vi "G# - CreatingAndDestroyingNamedObjects.vi"() -> ()   [LabVIEW 2020]
doc: "This example demonstrates how named objects work and also how objects behave if user counter is enabled.\n\nNaming Mode:\n1. Two objects with no names\n\nIf the object name is empty, a new object will always be created. User counter has no effect.\n\n2. Two objects with different names\n\nTwo objects are created with different name. There will be one user of each.\n\n3. Create and lookup object with equal names\n\nFirst a named object is created, then a new object with same name is attempted to be created, but since it already exists, the existing object with that name will be returned. If user counter is not enabled, create function will return error 400042. If user counter is enabled, the counter will be checked when trying to destroy the object and the object will not be destroyed until the last user of the object runs the destroy method."
uses:
  MyG#SubClass_class/MyG#SubClass.lvclass
  vi.lib/addons/_AddQ/G#Object/G#Object.lvclass
panel:
  out "# of objects killed":i32
  out "OK":bool
  in  "error in":errorcluster
  out "nr of users of the object":i32[](array[numeric])
  out "nr of objects of the class":i32[](array[numeric])
  in  "user counter":bool=TRUE
  in  "Naming mode":T1(ring)
  out "objects names":string[](array[string])
  out "error out":errorcluster
  # "This example demonstrates how named objects work and also how objects behave if user counter is enabled.\n\nNaming Mode:\n1. Two objects with no names\n\nIf the object name is empty, a new object will always be created. User counter has no effect.\n\n2. Two objects with different names\n\nTwo objects are created with different name. There will be one user of each.\n\n3. Create and lookup object with equal names\n\nFirst a named object is created, then a new object with same name is attempted to be created, but since it already exists, the existing object with that name will be returned. If user counter is not enabled, create function will return error 400042. If user counter is enabled, the counter will be checked when trying to destroy the object and the object will not be destroyed until the last user of the object runs the destroy method."
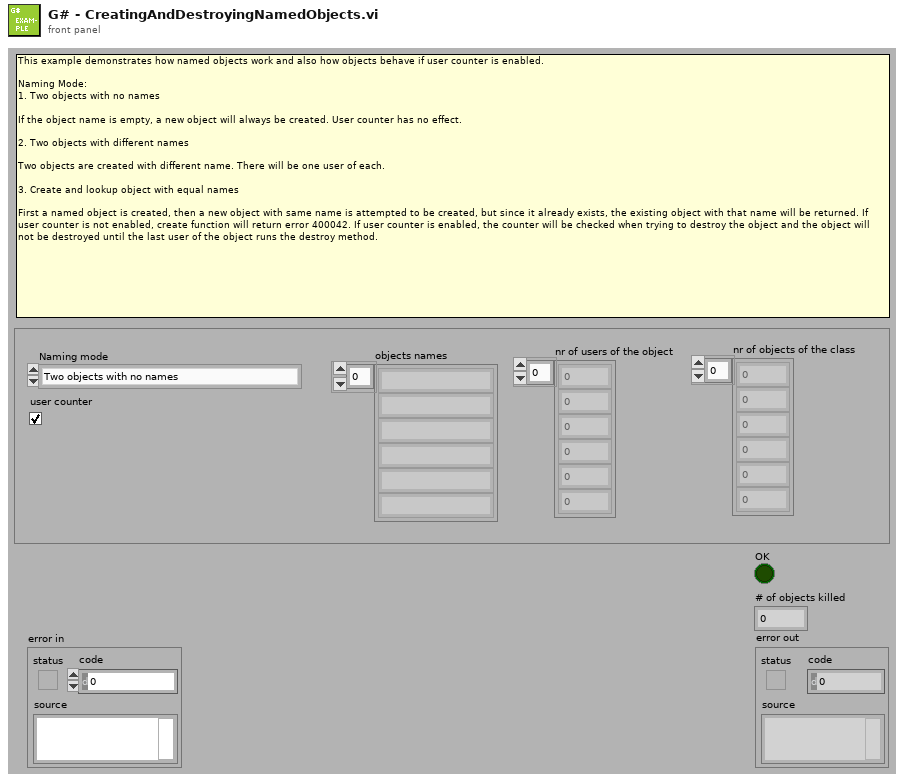
[diagram p1: front panel]
types:
  T1 = enum16{"Two objects with no names", "Two objects with different names", "Create and lookup object with equal names"}
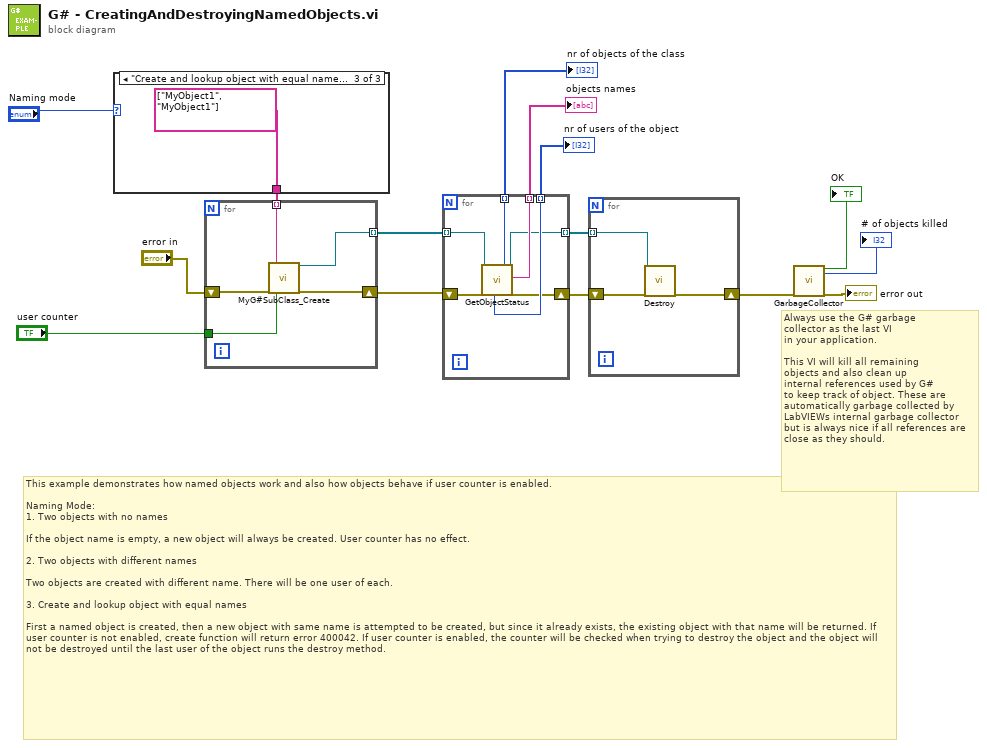
[diagram p0: block diagram]
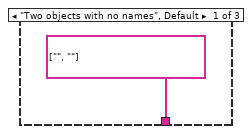
[diagram p2: hidden frame]
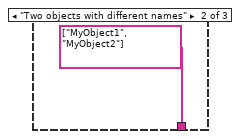
[diagram p3: hidden frame]
diagram:
  # "This example demonstrates how named objects work and also how objects behave if user counter is enabled.\n\nNaming Mode:\n1. Two objects with no names\n\nIf the object name is empty, a new object will always be created. User counter has no effect.\n\n2. Two objects with different names\n\nTwo objects are created with different name. There will be one user of each.\n\n3. Create and lookup object with equal names\n\nFirst a named object is created, then a new object with same name is attempted to be created, but since it already exists, the existing object with that name will be returned. If user counter is not enabled, create function will return error 400042. If user counter is enabled, the counter will be checked when trying to destroy the object and the object will not be destroyed until the last user of the object runs the destroy method."
  # "Always use the G# garbage\ncollector as the last VI\nin your application.\n\nThis VI will kill all remaining\nobjects and also clean up\ninternal references used by G#\nto keep track of object. These are\nautomatically garbage collected by\nLabVIEWs internal garbage collector\nbut is always nice if all references are\nclose as they should."
  n1 = case shown="\"Create and lookup object with equal names\"" "Naming mode" {
    tunnel: [string[] ["", ""] string[] ["MyObject1", "MyObject2"] string[] ["MyObject1", "MyObject1"]] -> w13
    frame "Two objects with no names", Default {
    }
    frame "Two objects with different names" {
    }
    frame "Create and lookup object with equal names" {
    }
  }
  n2 = for {
    shift-right: [w23] -> w9
    shift-left: "error in" -> [w22]
    tunnel: [w21] -> w15 mode=indexing
    tunnel: w13 -> [w20] mode=indexing
    tunnel: "user counter" -> [w19]
    n3 = call "MyG#SubClass_Create.vi"("error in (no error)"=w22, "object name"=w20, "user counter"=w19) -> ("reference out"=w21:refnum<class "MyG#SubClass.lvclass">, "error out"=w23:errorcluster)  [unwired: 15 in]
  }
  n4 = for {
    shift-right: [w25] -> w5
    shift-left: w9 -> [w30]
    tunnel: w15 -> [w29] mode=indexing
    tunnel: [w28] -> w8 mode=indexing
    tunnel: [w27] -> w7 mode=indexing
    tunnel: [w26] -> w6 mode=indexing
    tunnel: [w24] -> w3 mode=indexing
    n5 = call-dynamic "GetObjectStatus.vi"("reference in"=w29, "error in (no error)"=w30) -> ("# of users?"=w26:i32, "# of objects"=w28:i32, "reference out"=w24:refnum<class "MyG#SubClass.lvclass">, "object name"=w27:string, "error out"=w25:errorcluster)  [unwired: 6 in, 7 out]
  }
  "objects names" <- w7
  "nr of objects of the class" <- w8
  "nr of users of the object" <- w6
  n6 = for {
    shift-right: [w32] -> w4
    shift-left: w5 -> [w33]
    tunnel: w3 -> [w31] mode=indexing
    n7 = call-dynamic "Destroy.vi"("reference in"=w31, "error in (no error)"=w33) -> ("error out"=w32:errorcluster)  [unwired: 16 in, 1 out]
  }
  n8 = call "GarbageCollector.vi"("error in (no error)"=w4) -> ("OK"=→"OK":bool, "# of objects killed"=→"# of objects killed":i32, "error out"=→"error out":errorcluster)  [unwired: 16 in]
